vi "_RT Open Preference File.vi"(4 "error In":errorcluster) -> (0 "error":errorcluster, 3 "refnum":T1)   [LabVIEW 2015]
uses:
  <vilib>/Utility/config.llb/Config Data RefNum.ctl
  <vilib>/Utility/config.llb/NI_LVConfig.lvlib
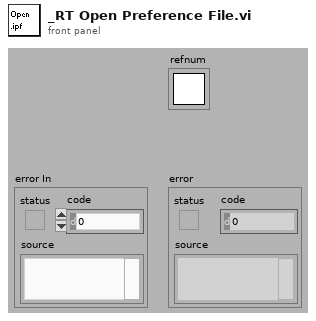
[diagram p1: front panel]
types:
  T1 = typedef "NI_LVConfig.lvlib/Config Data RefNum.ctl" = refnum<k1>
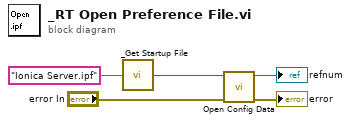
[diagram p0: block diagram]
diagram:
  n1 = call "_Get Startup File.vi"("FileName"="Ionica Server.ipf") -> ("FilePath"=w3:path)
  n2 = call <vilib>:"Open Config Data.vi"("error in (no error)"="error In", "configuration file path"=w3) -> ("error out"=→"error":errorcluster, "refnum"=→"refnum":T1)  [unwired: 7 in, 1 out]
